vi "add scan gating(SubVI).vi"(10 "字符串":string) -> (0 "布尔 3":bool, 2 "连接的字符串":string)   [LabVIEW 2019, in "Add Seq.lvlib"]
uses:
  Add Seq.lvlib
panel:
  in  "Number of Step":i32=19 min=0 max=70001
  in  "Step Delay(secs)":dbl
  in  "Gating ch(2614)":i32(ring) items=["ChA", "ChB"]
  in  "Increments(V)":dbl=1.0
  in  "cancel":bool
  in  "ok":bool
  in  "Rate(mV/s)":dbl=10.0
  in  "Final Voltage(V)":dbl=20.0 min=2.0 max=325.0
  in  "Initial Voltage(V)":dbl=2.0 min=2.0 max=325.0
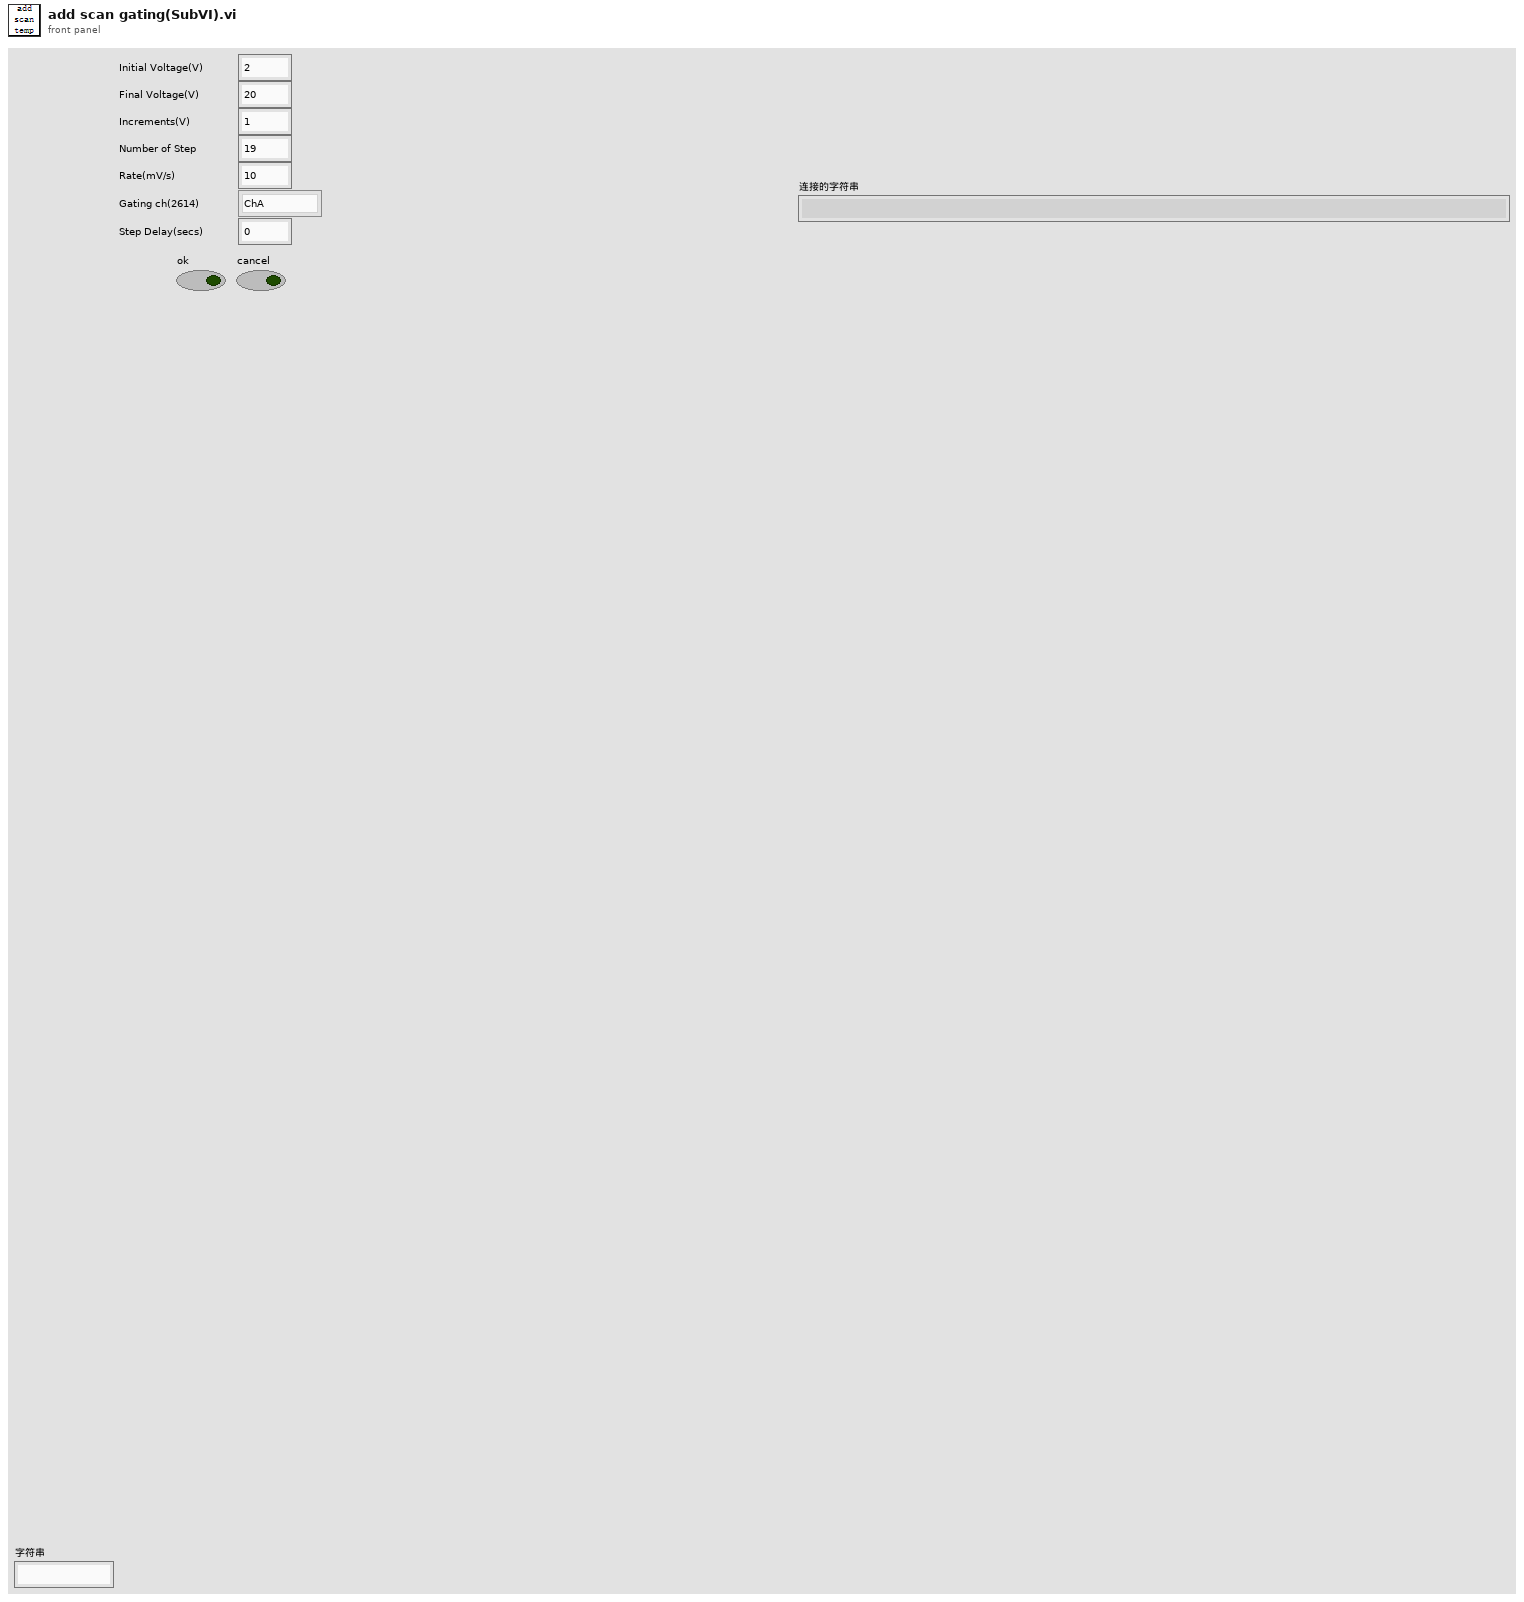
[diagram p1: front panel]
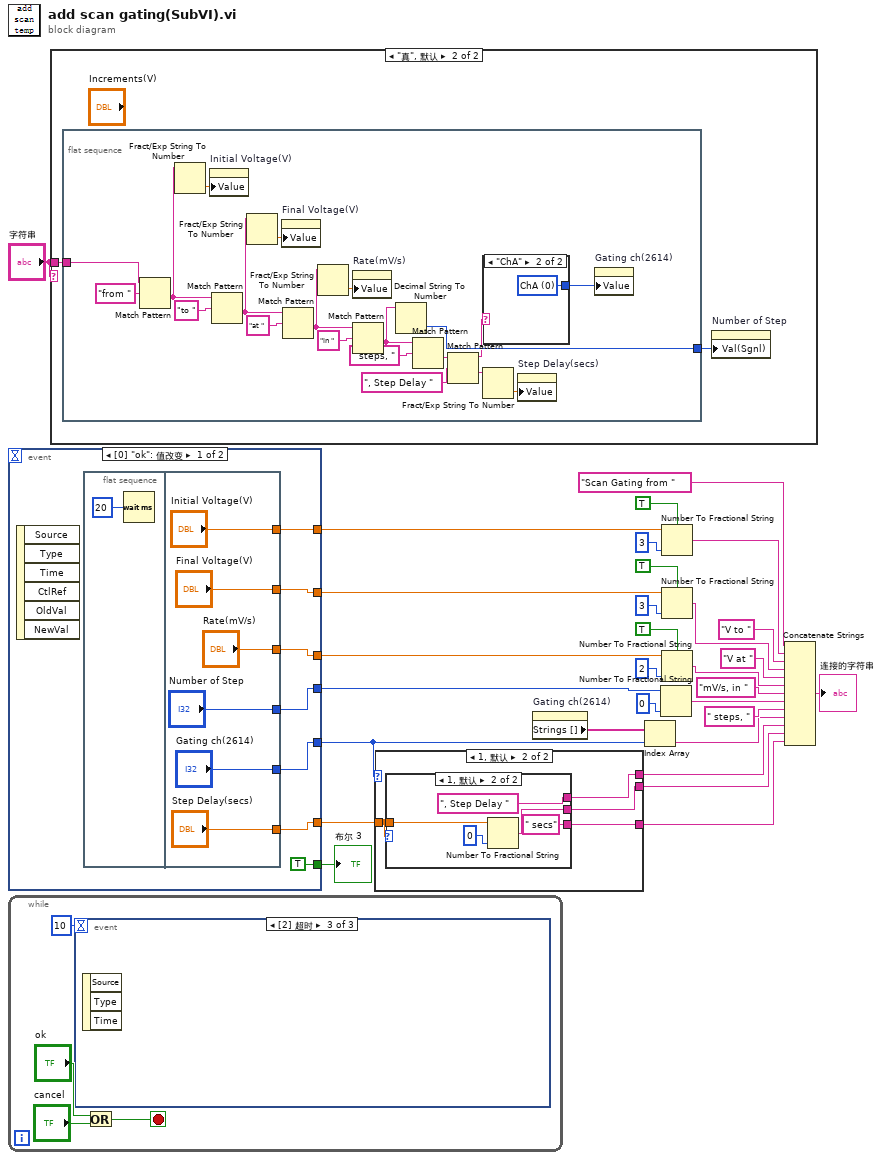
[diagram p0: block diagram]
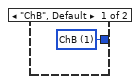
[diagram p3: hidden frame]
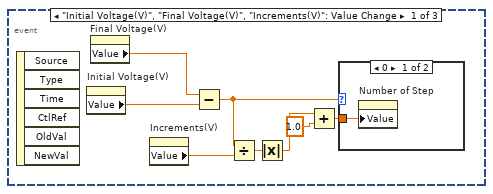
[diagram p4: hidden frame]
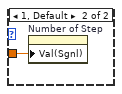
[diagram p5: hidden frame]
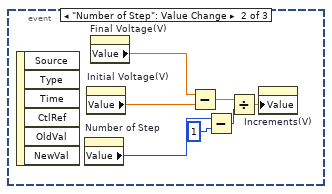
[diagram p6: hidden frame]
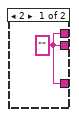
[diagram p7: hidden frame]
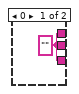
[diagram p8: hidden frame]
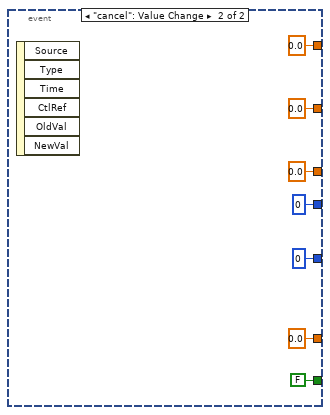
[diagram p9: hidden frame]
diagram:
  n1 = event shown="[0] \"ok\": 值改变" {
    selector: _ -> [_ _]
    dyn-events: _ -> [_ _]
    timeout: _ -> [_ _]
    tunnel: [w37 0.0 ("Field 2")] -> w19
    tunnel: [w36 0.0 ("Rate输入")] -> w16
    tunnel: [w35 0.0 ("Field")] -> w28
    tunnel: [TRUE FALSE] -> w30
    tunnel: [w31 0 ("Number of Step")] -> w13
    tunnel: [w33 0 ("Approach输入")] -> w5
    tunnel: [w32 0.0 ("Step Delay(secs)")] -> w6
    event "ok": Value Change {
      n2 = event-data() -> ()  [unwired: 1 in, 6 out]
      n3 = flat-sequence {
        tunnel: ["Final Voltage(V)"] -> w37
        tunnel: ["Rate(mV/s)"] -> w36
        tunnel: ["Initial Voltage(V)"] -> w35
        tunnel: ["Gating ch(2614)"] -> w33
        tunnel: ["Step Delay(secs)"] -> w32
        tunnel: ["Number of Step"] -> w31
        frame #0 {
          n4 = Wait (ms)(milliseconds to wait=u32 20 ("等待时间（毫秒）")) -> ()  [unwired: 1 out]
        }
        frame #1 {
        }
      }
    }
    event "cancel": Value Change {
      n5 = event-data() -> ()  [unwired: 1 in, 6 out]
    }
  }
  "布尔 3" <- w30
  n6 = while {
    stop <- w52 stop-if-true
    n7 = event shown="[2] 超时" {
      selector: _ -> [_ _ _]
      dyn-events: _ -> [_ _ _]
      timeout: 10 -> [_ _ _]
      event "Initial Voltage(V)", "Final Voltage(V)", "Increments(V)": Value Change {
        n8 = event-data() -> ()  [unwired: 1 in, 6 out]
        n9 = property on="Initial Voltage(V)" class="DigNum (严格)"() -> ("Value"=w63:dbl)  [unwired: 2 in, 2 out]
        n10 = property on="Final Voltage(V)" class="DigNum (严格)"() -> ("Value"=w58:dbl)  [unwired: 2 in, 2 out]
        n11 = property on="Increments(V)" class="DigNum (严格)"() -> ("Value"=w62:dbl)  [unwired: 2 in, 2 out]
        n12 = Subtract(x=w58, y=w63) -> (x-y=w57:dbl)
        n13 = Divide(x=w57, y=w62) -> (x/y=w60:dbl)
        n14 = Absolute Value(x=w60) -> (abs(x)=w59:dbl)
        n15 = Add(x=w59, y=1.0) -> (x+y=w56:dbl)
        n16 = case shown="0" w57 {
          tunnel: w56 -> [w64 w65]
          frame 0 {
            n17 = property on="Number of Step" class="DigNum (严格)"("Value"=w64) -> ()  [unwired: 2 in, 2 out]
          }
          frame 1, Default {
            n18 = property on="Number of Step" class="DigNum (严格)"("Val(Sgnl)"=w65) -> ()  [unwired: 2 in, 2 out]
          }
        }
      }
      event "Number of Step": Value Change {
        n19 = event-data() -> ()  [unwired: 1 in, 6 out]
        n20 = property on="Number of Step" class="DigNum (严格)"() -> ("Value"=w69:i32)  [unwired: 2 in, 2 out]
        n21 = property on="Initial Voltage(V)" class="DigNum (严格)"() -> ("Value"=w71:dbl)  [unwired: 2 in, 2 out]
        n22 = property on="Final Voltage(V)" class="DigNum (严格)"() -> ("Value"=w72:dbl)  [unwired: 2 in, 2 out]
        n23 = Subtract(x=w72, y=w71) -> (x-y=w70:dbl)
        n24 = Subtract(x=w69, y=1) -> (x-y=w67:i32)
        n25 = Divide(x=w70, y=w67) -> (x/y=w66:dbl)
        n26 = property on="Increments(V)" class="DigNum (严格)"("Value"=w66) -> ()  [unwired: 2 in, 2 out]
      }
      event Timeout {
        n27 = event-data() -> ()  [unwired: 1 in, 3 out]
      }
    }
    n28 = Or(x="ok", y="cancel") -> (x .or. y?=w52:bool)
  }
  n29 = case shown="\"真\", 默认" "字符串" {
    tunnel: "字符串" -> [_ w73]
    frame "" {
    }
    frame "真", Default {
      n30 = flat-sequence {
        tunnel: [w80] -> w74
        tunnel: w73 -> [w88]
        frame #0 {
          n31 = Match Pattern(string=w88, regular expression="from " ("正则表达式")) -> (after substring=w86:string)  [unwired: 1 in, 3 out]
          n32 = Fract/Exp String To Number(string=w86) -> (number=w90:dbl)  [unwired: 3 in, 1 out]
          n33 = property on="Initial Voltage(V)" class="DigNum (严格)"("Value"=w90) -> ()  [unwired: 2 in, 2 out]
          n34 = Match Pattern(string=w86, regular expression="to " ("正则表达式")) -> (after substring=w85:string)  [unwired: 1 in, 3 out]
          n35 = Fract/Exp String To Number(string=w85) -> (number=w91:dbl)  [unwired: 3 in, 1 out]
          n36 = property on="Final Voltage(V)" class="DigNum (严格)"("Value"=w91) -> ()  [unwired: 2 in, 2 out]
          n37 = Match Pattern(string=w85, regular expression="at " ("正则表达式")) -> (after substring=w82:string)  [unwired: 1 in, 3 out]
          n38 = Fract/Exp String To Number(string=w82) -> (number=w83:dbl)  [unwired: 3 in, 1 out]
          n39 = property on="Rate(mV/s)" class="DigNum (严格)"("Value"=w83) -> ()  [unwired: 2 in, 2 out]
          n40 = Match Pattern(string=w82, regular expression="in " ("正则表达式")) -> (after substring=w79:string)  [unwired: 1 in, 3 out]
          n41 = Decimal String To Number(string=w79) -> (number=w80:i32)  [unwired: 2 in, 1 out]
          n42 = Match Pattern(string=w79, regular expression=" steps, " ("正则表达式")) -> (after substring=w77:string)  [unwired: 1 in, 3 out]
          n43 = Match Pattern(string=w77, regular expression=", Step Delay ") -> (before substring=w76:string, after substring=w94:string)  [unwired: 1 in, 2 out]
          n44 = case shown="\"ChA\"" w76 {
            tunnel: [w95 w96] -> w75
            frame "ChB", Default {
              w95 = 1 items=["ChA", "ChB"] ("Gating ch(2614)")
            }
            frame "ChA" {
              w96 = 0 items=["ChA", "ChB"] ("Gating ch(2614)")
            }
          }
          n45 = Fract/Exp String To Number(string=w94) -> (number=w92:dbl)  [unwired: 3 in, 1 out]
          n46 = property on="Step Delay(secs)" class="DigNum (严格)"("Value"=w92) -> ()  [unwired: 2 in, 2 out]
          n47 = property on="Gating ch(2614)" class="Ring (严格)"("Value"=w75) -> ()  [unwired: 2 in, 2 out]
        }
      }
      n48 = property on="Number of Step" class="DigNum (严格)"("Val(Sgnl)"=w74) -> ()  [unwired: 2 in, 2 out]
    }
  }
  n49 = case shown="1, 默认" w5 {
    tunnel: [w97 w101] -> w4
    tunnel: [w97 w100] -> w2
    tunnel: w6 -> [_ w98]
    tunnel: [w97 w99] -> w3
    frame 2 {
      w97 = ""
    }
    frame 1, Default {
      n50 = case shown="1, 默认" w98 {
        tunnel: [w102 ", Step Delay " ("字符串")] -> w101
        tunnel: [w102 " secs" ("字符串")] -> w100
        tunnel: w98 -> [_ w105]
        tunnel: [w102 w104] -> w99
        frame 0 {
          w102 = ""
        }
        frame 1, Default {
          n51 = Number To Fractional String(number=w105, precision (6)=i16 0 ("精度(6)")) -> (F-format string=w104:string)  [unwired: 2 in]
        }
      }
    }
  }
  n52 = property on="Gating ch(2614)" class="Ring (严格)"() -> ("Strings []"=w7:string[])  [unwired: 2 in, 2 out]
  n53 = Index Array(array=w7, index=w5) -> (element=w9:string)
  n54 = Number To Fractional String(number=w13, precision (6)=i16 0 ("精度(6)")) -> (F-format string=w12:string)  [unwired: 2 in]
  n55 = Number To Fractional String(use system decimal point (T)=TRUE ("使用系统小数点(T)"), number=w28, precision (6)=i16 3 ("精度(6)")) -> (F-format string=w26:string)  [unwired: 1 in]
  n56 = Number To Fractional String(use system decimal point (T)=TRUE ("使用系统小数点(T)"), number=w19, precision (6)=i16 3 ("精度(6)")) -> (F-format string=w21:string)  [unwired: 1 in]
  n57 = Number To Fractional String(use system decimal point (T)=TRUE ("使用系统小数点(T)"), number=w16, precision (6)=i16 2 ("精度(6)")) -> (F-format string=w15:string)  [unwired: 1 in]
  n58 = Concatenate Strings("Scan Gating from " ("字符串"), w26, "V to " ("字符串"), w21, "V at " ("字符串"), w15, "mV/s, in " ("字符串"), w12, " steps, " ("字符串"), w9, w4, w3, w2) -> (→"连接的字符串":string)
